vi "RIO Teams Folder Path.vi"() -> (2 "RIO Teams Folder":string="home/lvuser/TeamFiles", 3 "Teams Folder":path)   [LabVIEW 2020]
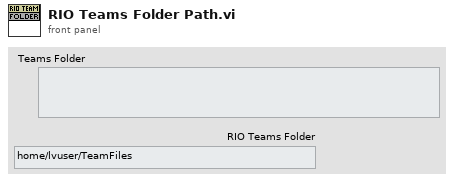
[diagram p1: front panel]
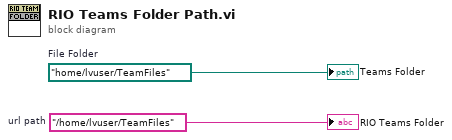
[diagram p0: block diagram]
diagram:
  w1 = "/home/lvuser/TeamFiles"  # url path
  w2 = path "/home/lvuser/TeamFiles"  # File Folder
  "Teams Folder" <- w2
  "RIO Teams Folder" <- w1
